vi "poly_lock_fp_updates_unlock_self.vi"(8 "error in":errorcluster) -> (0 "error out":errorcluster)   [LabVIEW 2015]
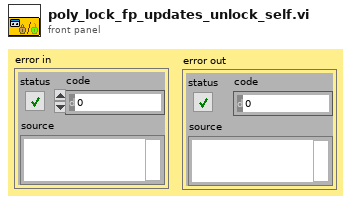
[diagram p1: front panel]
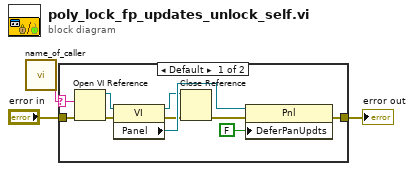
[diagram p0: block diagram]
diagram:
  n1 = call "name_of_caller.vi"() -> ("name of caller out"=w1:string)  [unwired: 4 in]
  n2 = case shown="Default" w1 {
    selector: w1 -> [w10 _]
    tunnel: [w12 w14] -> w3
    tunnel: "error in" -> [w9 w14]
    frame Default {
      n3 = Open VI Reference(vi path=w10, error in (no error)=w9) -> (vi reference=w7:refnum<vi>, error out=w8:errorcluster)  [unwired: 4 in]
      n4 = property class="VI"(reference=w7, error in=w8) -> (reference out=w4:refnum<vi>, error out=w6:errorcluster, "Panel"=w11:refnum<vi>)
      n5 = Close Reference(reference=w4, error in (no error)=w6) -> (error out=w5:errorcluster)
      n6 = property class="Pnl"(reference=w11, error in=w5, "DeferPanUpdts"=FALSE) -> (error out=w12:errorcluster)  [unwired: 1 out]
    }
    frame "" {
    }
  }
  "error out" <- w3
